vi "Render.vi"(8 "error in (no error)":errorcluster, 10 "String in":string, 11 "Image in":refnum<class "Image.lvclass">) -> (0 "error out":errorcluster, 2 "String out":string, 3 "Image out":refnum<class "Image.lvclass">)   [LabVIEW 2021, in "LvMarkdown.lvlib" / "Image.lvclass"]
uses:
  Image.lvclass
  Image.lvclass/Image.ctl
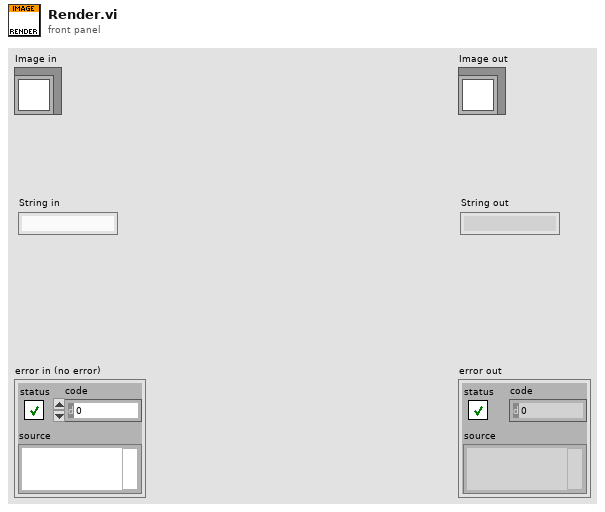
[diagram p1: front panel]
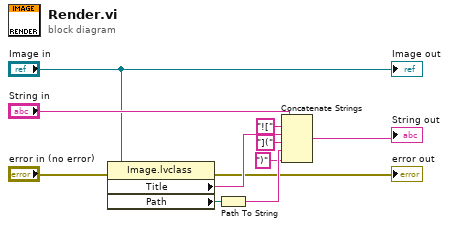
[diagram p0: block diagram]
diagram:
  n1 = property class="Image.lvclass"(reference="Image in", error in="error in (no error)") -> (error out=→"error out":errorcluster, "Title"=w8:string, "Path"=w3:path)  [unwired: 1 out]
  n2 = Path To String(path=w3) -> (string=w6:string)
  n3 = Concatenate Strings("String in", "![" ("string"), w8, "](" ("string"), w6, ")" ("string")) -> (→"String out":string)
  "Image out" <- "Image in"
